vi "ReadFromCSV.vi"() -> ()   [LabVIEW 2019]
uses:
  <vilib>/Utility/file.llb/Read Delimited Spreadsheet (DBL).vi
  <vilib>/Utility/file.llb/Read Delimited Spreadsheet (string).vi
panel:
  out "all rows 2":dbl[][](array[numeric])
  out "appended path 2":path
  out "appended path":path
  out "text":string
  out "all rows":string[][](array[string])
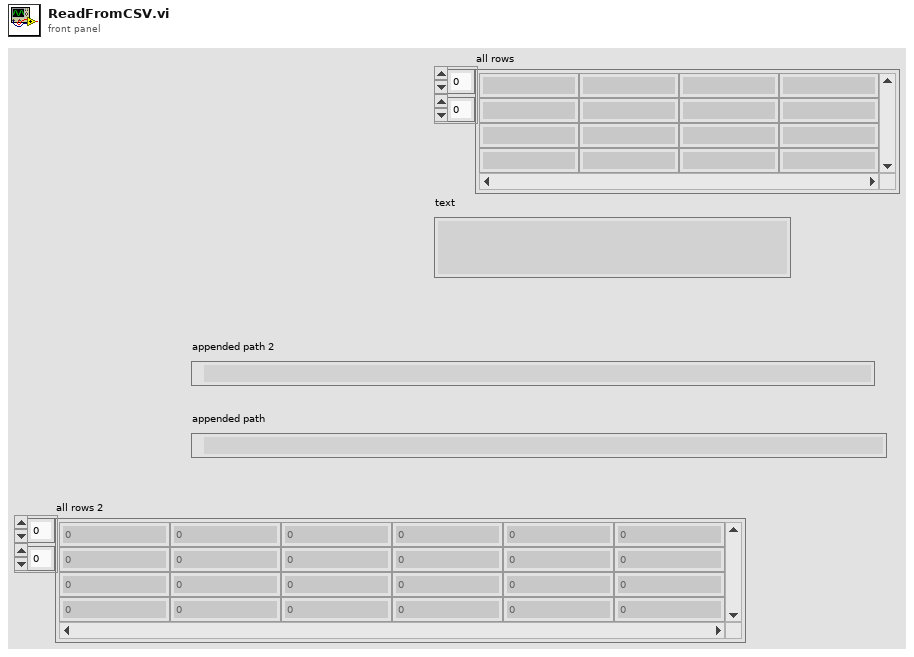
[diagram p1: front panel]
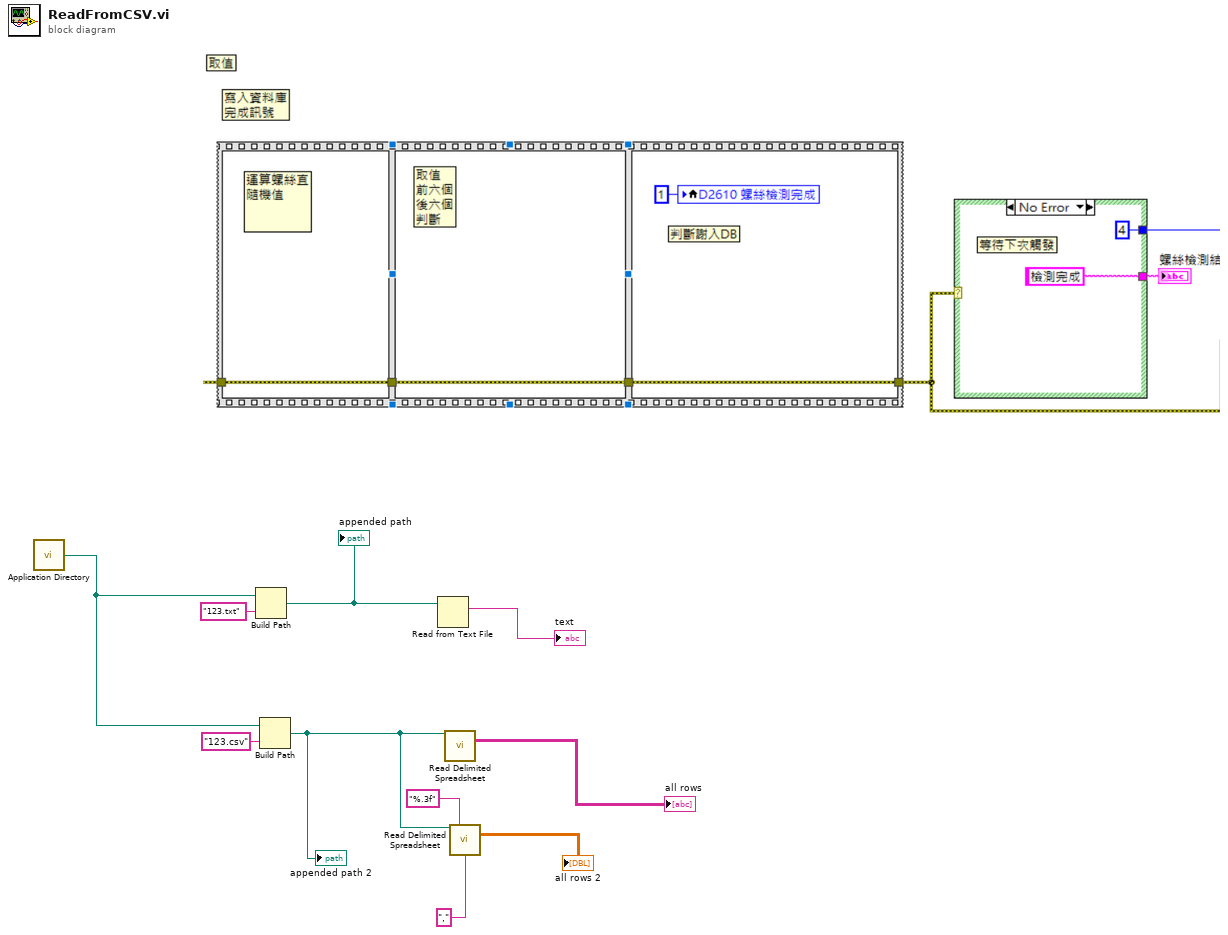
[diagram p0: block diagram]
diagram:
  n1 = call <vilib>:"Application Directory.vi"() -> ("Application Directory"=w8:path)
  n2 = Build Path(base path=w8, name or relative path="123.txt") -> (appended path=w7:path)
  "appended path" <- w7
  n3 = Build Path(base path=w8, name or relative path="123.csv") -> (appended path=w4:path)
  "appended path 2" <- w4
  n4 = Read from Text File(file (use dialog)=w7) -> (text=→"text":string)  [unwired: 3 in, 3 out]
  n5 = call-poly <vilib>:"Read Delimited Spreadsheet.vi"("file path (dialog if empty)"=w4) -> ("all rows"=→"all rows":string[][])  [unwired: 9 in, 5 out]
  n6 = call-poly <vilib>:"Read Delimited Spreadsheet.vi"("file path (dialog if empty)"=w4, "format (%.3f)"="%.3f", "delimiter (\\t)"="," ("delimiter (\\t)")) -> ("all rows"=→"all rows 2":dbl[][])  [unwired: 7 in, 5 out]
